vi "Calculate Increment.vi"(7 "LBCB Number":T1, 8 "Increment Limits":T6, 9 "Previous":T6, 10 "Current":T6, 11 "Within Limits In":T2) -> (1 "Limit Fault":bool, 3 "Within Limits Out":T2)   [LabVIEW 2009]
uses:
  Control Loop/Act & Cart Commands.ctl
  Within Limits Matrix.ctl
  Actuator Faults.ctl
  Cart Disp Faults.ctl
  Cart Force Faults.ctl
  Data Access Objects/Metadata/LBCB Number.ctl
  Data Access Objects/Metadata/DAO Actions.ctl
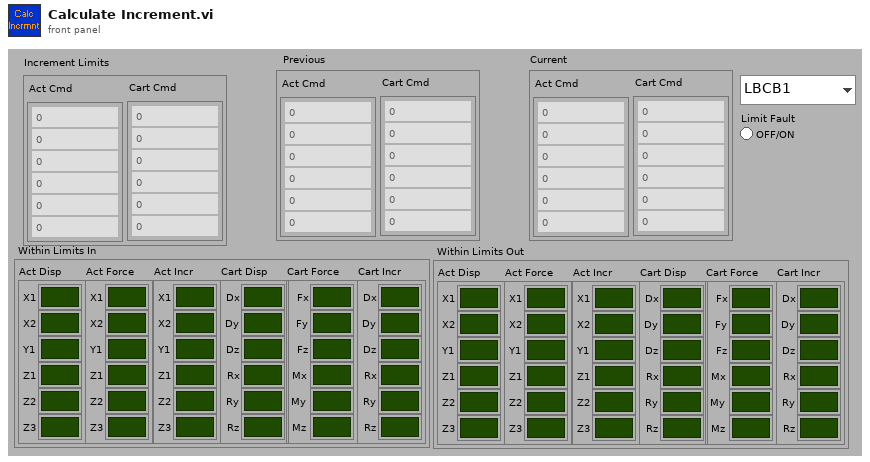
[diagram p1: front panel]
types:
  T1 = typedef "LBCB Number.ctl" = enum16{"LBCB1", "LBCB2"}
  T2 = typedef "Within Limits Matrix.ctl" = cluster{"Act Disp":T3, "Act Force":T3, "Act Incr":T3, "Cart Disp":T4, "Cart Force":T5, "Cart Incr":T4}
  T3 = typedef "Actuator Faults.ctl" = cluster{"X1":bool, "X2":bool, "Y1":bool, "Z1":bool, "Z2":bool, "Z3":bool}
  T4 = typedef "Cart Disp Faults.ctl" = cluster{"Dx":bool, "Dy":bool, "Dz":bool, "Rx":bool, "Ry":bool, "Rz":bool}
  T5 = typedef "Cart Force Faults.ctl" = cluster{"Fx":bool, "Fy":bool, "Fz":bool, "Mx":bool, "My":bool, "Mz":bool}
  T6 = typedef "Act & Cart Commands.ctl" = cluster{"Act Cmd":dbl[], "Cart Cmd":dbl[]}
  T7 = typedef "DAO Actions.ctl" = enum16{"Init", "Get", "Set"}
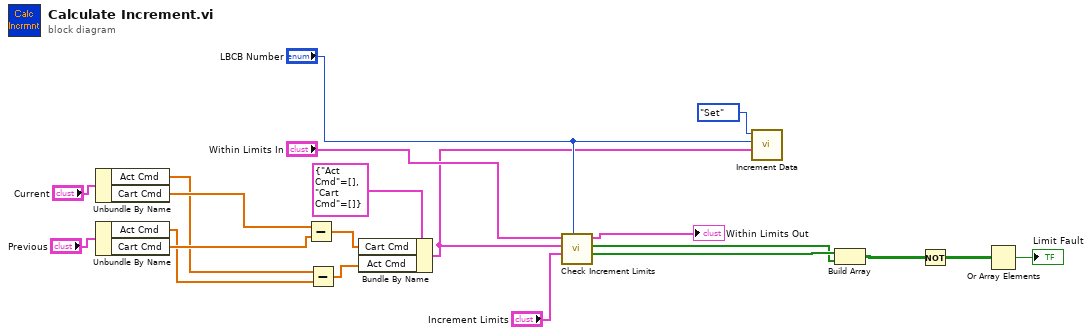
[diagram p0: block diagram]
diagram:
  n1 = Unbundle By Name("Current") -> ("Act Cmd"=w8:dbl[], "Cart Cmd"=w18:dbl[])
  n2 = Unbundle By Name("Previous") -> ("Act Cmd"=w7:dbl[], "Cart Cmd"=w17:dbl[])
  n3 = Subtract(x=w18, y=w17) -> (x-y=w3:dbl[])
  n4 = Subtract(x=w8, y=w7) -> (x-y=w2:dbl[])
  n5 = Bundle By Name(cluster=T6 {"Act Cmd"=[], "Cart Cmd"=[]} ("Increments In"), "Cart Cmd"=w3, "Act Cmd"=w2) -> (w1:T6)
  n6 = call "Check Increment Limits.vi"("LBCB Number"="LBCB Number", "Increment Limits"="Increment Limits", "Increments In"=w1, "Within Limits In"="Within Limits In") -> ("Cartesian In Limit"=w13:bool[], "Actuator In Limit"=w4:bool[], "Within Limits Out"=→"Within Limits Out":T2)  [unwired: 2 in, 1 out]
  n7 = call "Increment Data.vi"("Increments In"=w1, "LBCB Number"="LBCB Number", "DAO Actions"=DAO_Actions."Set") -> ()  [unwired: 7 in, 2 out]
  n8 = Build Array(w13, w4) -> (w6:bool[][])
  n9 = Not(x=w6) -> (.not. x?=w11:bool[][])
  n10 = Or Array Elements(Boolean array=w11) -> (logical OR=→"Limit Fault":bool)
